vi "imp_test_v11_p2.vi"() -> ()   [LabVIEW 2014]
uses:
  <vilib>/LabVIEW Targets/FPGA/cRIO/shared/nicrio_ModuleControls/nicrio_cRIO-9237_DataRatesRing.ctl
  <vilib>/LabVIEW Targets/FPGA/cRIO/shared/nicrio_ModuleControls/nicrio_cRIO-9237_ExcitationVoltageRing.ctl
  <vilib>/rvi/FXPMathLib/FxpSinAndCos/subVIs/nifxpmath_SinAndCos_SimConfig.ctl
  <vilib>/rvi/Emulation/niFpgaGetClockAttributes.vi
  <vilib>/rvi/Emulation/niFpgaSctlEmulationGetInTimedLoop.vi
  <vilib>/rvi/Emulation/niFpgaEmulationReportErrorSimple.vi
  <vilib>/rvi/Emulation/niFpgaProcessEmulError.vi
  <vilib>/rvi/interface/RandomDataEmulation/nirviRandomDataMultiElementFPGAFIFO.vi
  <instcachedir>/0/nirviRandomDataMultiElementFPGAFIFO_AD0CFC12EF974623A9C2E4184BC062B2.lvgen/nirviRandomDataMultiElementFPGAFIFO_AD0CFC12EF974623A9C2E4184BC062B2_028.vi
  <vilib>/rvi/interface/RandomDataEmulation/niFpgaRandomDataHandleErrors.vi
  <vilib>/rvi/Emulation/niFpgaCriticalErrorInLSC.vi
  <vilib>/rvi/FXPMathLib/FxpSinAndCos/simVIs/DllFxpSinAndCosTemp_sub.vi
  <vilib>/rvi/eio/common/nirviEmuTemplateMethod_errors.vi
  <vilib>/rvi/eio/common/nirviEmuTemplatePropertySet_errors.vi
  <vilib>/rvi/DataTransferAndStorage/Container/XNode/niFpgaContainer.xnode
  <vilib>/rvi/interface/RandomDataEmulation/nirviRandomDataFpgaMultiElementTemplate.vi
  <vilib>/rvi/Analysis/measure/butterworth/XNode/niFpgaButterworthFilter.xnode
  <vilib>/rvi/FXPMathLib/FxpSinAndCos/XNode/nifxpmath_SinAndCos.xnode
  <vilib>/eio/EIONode/EIONode.xnode
  <vilib>/eio/EIOPropertyNode/EIOPropertyNode.xnode
  <vilib>/rvi/eio/common/nirviEmuTemplatePropertyGet_errors.vi
  <vilib>/rvi/eio/common/nirviEmuTemplatePropertyGet_noerrors.vi
  <vilib>/rvi/eio/common/nirviEmuTemplatePropertySet_noerrors.vi
panel:
  in  "Mavg f loop(uSec)":u32
  in  "F_Threshold_p":fxp<+,12,4>
  out "omega_p (Mavg)":fxp<+/-,36,13>
  out "Dp_d (Mavg)":fxp<+/-,36,13>
  out "omega_p2 (Mavg)":fxp<+/-,36,14>
  out "Dp2_d (Mavg)":fxp<+/-,36,14>
  in  "mt0_p2":u32
  out "Dp_d (Mavg w. f.)":fxp<+/-,36,14>
  in  "Dp_d (Mavg) coeff.":i32[](array[numeric])=[946630756, 63555534]
  out "omega_p (Mavg w. f)":fxp<+/-,36,14>
  in  "omega_P(Mavg) coeff.":i32[](array[numeric])=[946630756, 63555534]
  out "PID (kHz)":fxp<+/-,20,10>
  in  "Set 6":bool
  in  "Set 5":bool
  in  "Set 4":bool
  in  "Set 3":bool
  in  "Set 2":bool
  in  "Set 1":bool
  out "Dp1_d (T)":fxp<+/-,36,13>
  out "omega_p1 (T)":fxp<+/-,36,13>
  out "Dp2_d (T)":fxp<+/-,36,13>
  out "omega_p2 (T)":fxp<+/-,36,13>
  out "mt_omega_p2":u32
  out "Encoder Position_p2":i32
  out "D_p2":fxp<+/-,32,7>
  out "rad_p2":fxp<+/-,33,20>
  out "D_p1":fxp<+/-,32,7>
  out "rad_p1":fxp<+/-,33,20>
  out "Encoder Position_p1":i32
  out "Dp1_d (Mavg)":fxp<+/-,36,14>
  out "omega_p1 (Mavg)":fxp<+/-,36,14>
  in  "Dp_d_M_avg_Tc (uSec)":i32
  out "Dp_d (T)":fxp<+/-,36,13>
  out "omega_p (T)":fxp<+/-,36,13>
  in  "Vp. Est.":i16(ring) items=["T", "Mavg", "Mavg w. f."]
  in  "Mag. factor_p":fxp<+/-,20,3>
  in  "Mag. encoder_p":bool
  in  "Belt_out_p":fxp<+/-,7,7>
  in  "Belt_in_p":fxp<+/-,6,6>
  out "Fp_dc":fxp<+/-,32,10>
  in  "Zero_p":bool
  in  "mt0_p1":u32
  in  "Encoder reset":bool
  out "fpt_d":fxp<+/-,36,18>
  out "Dp_error_dd":fxp<+/-,36,16>
  out "Dp_error_d":fxp<+/-,33,8>
  in  "Dp_dd coeff.":i32[](array[numeric])=[946630756, 63555534]
  out "Dp_dd":fxp<+/-,36,25>
  out "dFp_PID":fxp<+/-,36,18>
  in  "dFp_PID coeff.":i32[](array[numeric])=[946630756, 63555534]
  out "fpt_i":fxp<+/-,34,18>
  in  "Bv_p":fxp<+/-,22,8>
  in  "Kv_p":fxp<+/-,26,7>
  out "Dp_error":fxp<+/-,22,7>
  out "Dpr_sin":fxp<+/-,22,7>
  in  "Sin offset_p":fxp<+/-,22,7>
  in  "Sin magnitude_p":fxp<+/-,21,6>
  out "Dpr_sin_dd":fxp<+/-,35,20>
  out "Dpr_sin_d":fxp<+/-,33,15>
  out "Sin omega_p":fxp<+/-,34,9>
  in  "Sin wave freq._p (Hz)":fxp<+/-,32,6>
  in  "Dpr_step":fxp<+/-,22,7>
  out "Dpr_for":fxp<+/-,22,7>
  in  "Command_p":i16(ring) items=["Step", "Sine"]
  in  "Ki_p":fxp<+/-,30,9>
  out "Fp_PID":fxp<+/-,36,16>
  in  "fp_tolorance":fxp<+,22,6>
  out "fp_tilde":fxp<+/-,33,10>
  in  "Kd_p":fxp<+/-,30,9>
  in  "Kp_p":fxp<+/-,32,13>
  out "Fr_p":fxp<+/-,32,10>
  in  "S/F coeff_p":fxp<+/-,25,-10>
  out "va_p":fxp<+/-,36,7>
  out "vb_p":fxp<+/-,37,8>
  out "vq_p_F":fxp<+/-,20,5> format="%.57g"
  out "vd_p_F":fxp<+/-,20,5>
  in  "dFp_add":bool
  in  "Stop motor_p":bool
  out "Force_p":fxp<+/-,32,10>
  in  "Strain selection_p":i16(ring) items=["Raw", "Avg.8", "Avg.8 w. filter"]
  out "Strain_p (Avg8 w. f)":fxp<+/-,36,8>
  in  "Strain_p Avg.8 coeff.":i32[](array[numeric])=[946630756, 63555534]
  out "Strain_p (Avg8)":fxp<+/-,36,4>
  out "Raw Strain_p":fxp<+/-,36,4>
  out "Mod6/AI3":fxp<+/-,36,4>
  in  "Strain gage reset_p":bool
  out "Dp_d (mm/s)":fxp<+/-,36,13>
  out "omega_p (rad/s)":fxp<+/-,36,13>
  out "mt_omega_p1":u32
  out "rad_p(NrTheta)":fxp<+/-,33,20>
  out "D_p(mm)":fxp<+/-,32,7>
  out "Encoder Position_p":i32
  in  "Encoder reset_p":bool
  out "Time now(s)":fxp<+,52,14>
  in  "Drive mode":i16(ring) items=["Backward", "Forward", "Imp"]
  in  "Ini coe.":bool
  out "Loop rate (kHz)":fxp<+/-,36,7>
  in  "Stop (Strain)":bool
  in  "Excitation Voltage":T1 items=["2.5 Volts", "3.3 Volts", "5.0 Volts", "10.0 Volts", "External Excitation"]
  in  "Data Rate":T2=1 items=["50.000 kS/s (NI 9237)"=1, "25.000 kS/s (NI 9237)"=2, "16.667 kS/s (NI 9237)"=3, "12.500 kS/s (NI 9237)"=4, "10.000 kS/s (NI 9237)"=5, "8.333 kS/s (NI 9237)"=6, "7.143 kS/s (NI 9237)"=7, "6.250 kS/s (NI 9237)"=8, "5.556 kS/s (NI 9237)"=9, "5.000 kS/s (NI 9237)"=10, "4.545 kS/s (NI 9237)"=11, "4.167 kS/s (NI 9237)"=12, "3.846 kS/s (NI 9237)"=13, "3.571 kS/s (NI 9237)"=14, "3.333 kS/s (NI 9237)"=15, "3.125 kS/s (NI 9237)"=16, "2.941 kS/s (NI 9237)"=17, "2.778 kS/s (NI 9237)"=18, "2.632 kS/s (NI 9237)"=19, "2.500 kS/s (NI 9237)"=20, "2.381 kS/s (NI 9237)"=21, "2.273 kS/s (NI 9237)"=22, "2.174 kS/s (NI 9237)"=23, "2.083 kS/s (NI 9237)"=24, "2.000 kS/s (NI 9237)"=25, "1.923 kS/s (NI 9237)"=26, "1.852 kS/s (NI 9237)"=27, "1.786 kS/s (NI 9237)"=28, "1.724 kS/s (NI 9237)"=29, "1.667 kS/s (NI 9237)"=30, "1.613 kS/s (NI 9237)"=31]
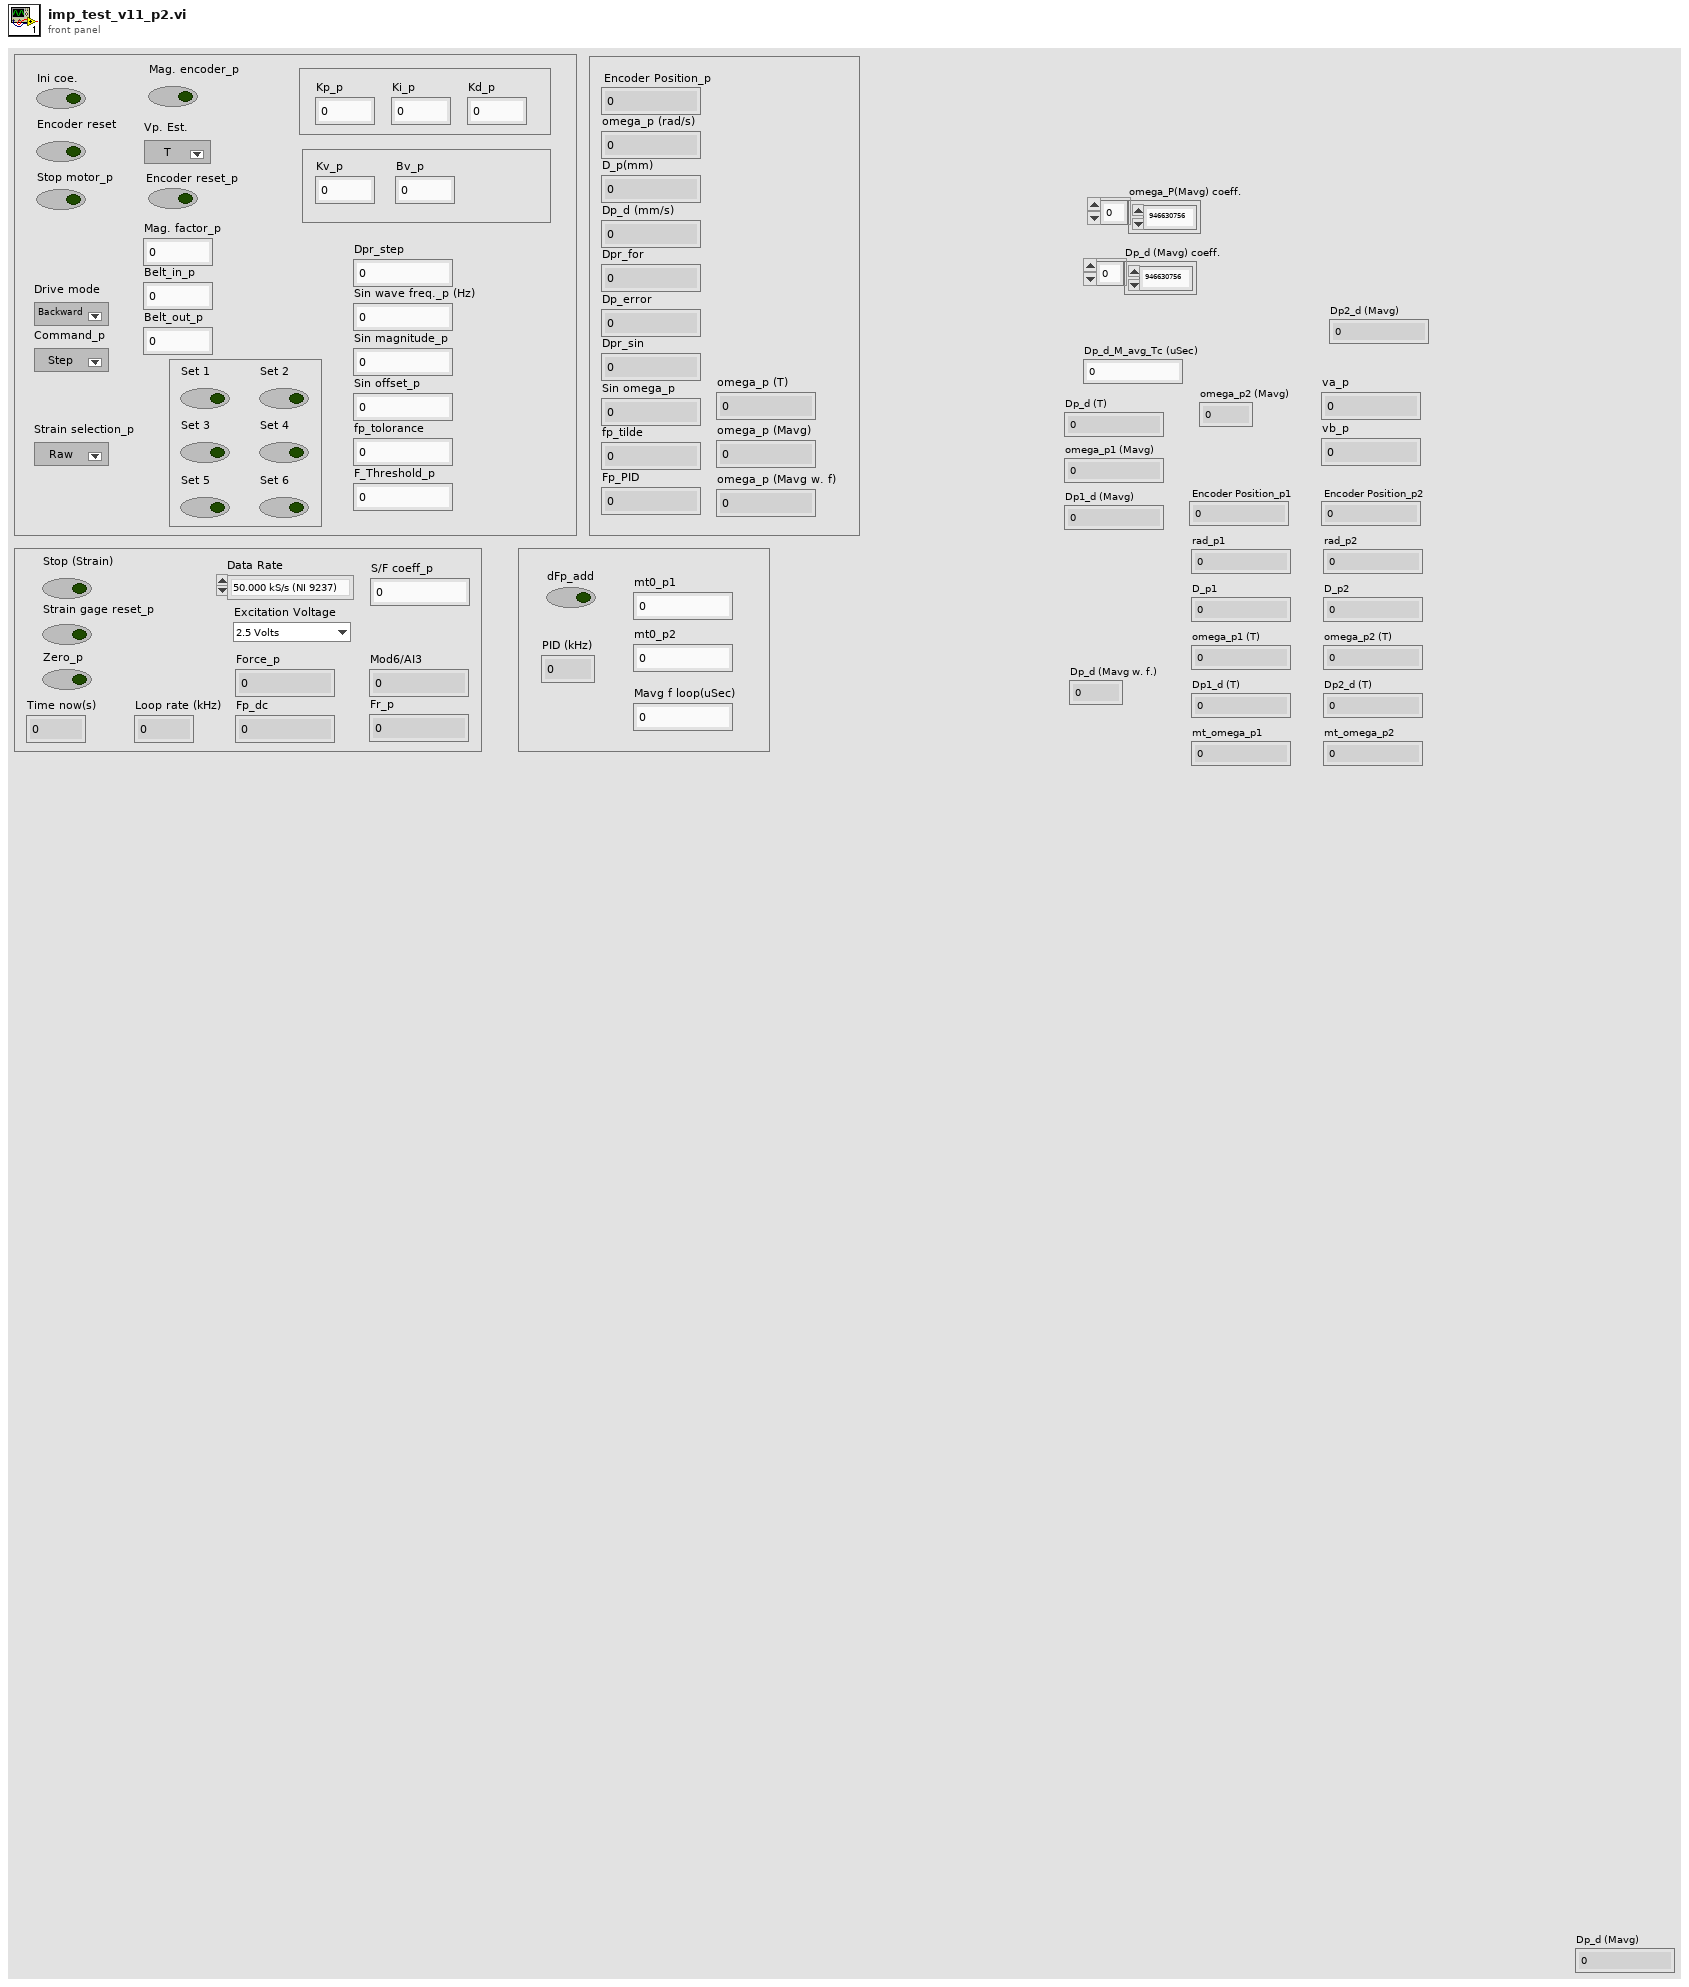
[diagram p1: front panel]
types:
  T1 = typedef "nicrio_cRIO-9237_ExcitationVoltageRing.ctl" = u8
  T2 = typedef "nicrio_cRIO-9237_DataRatesRing.ctl" = u8
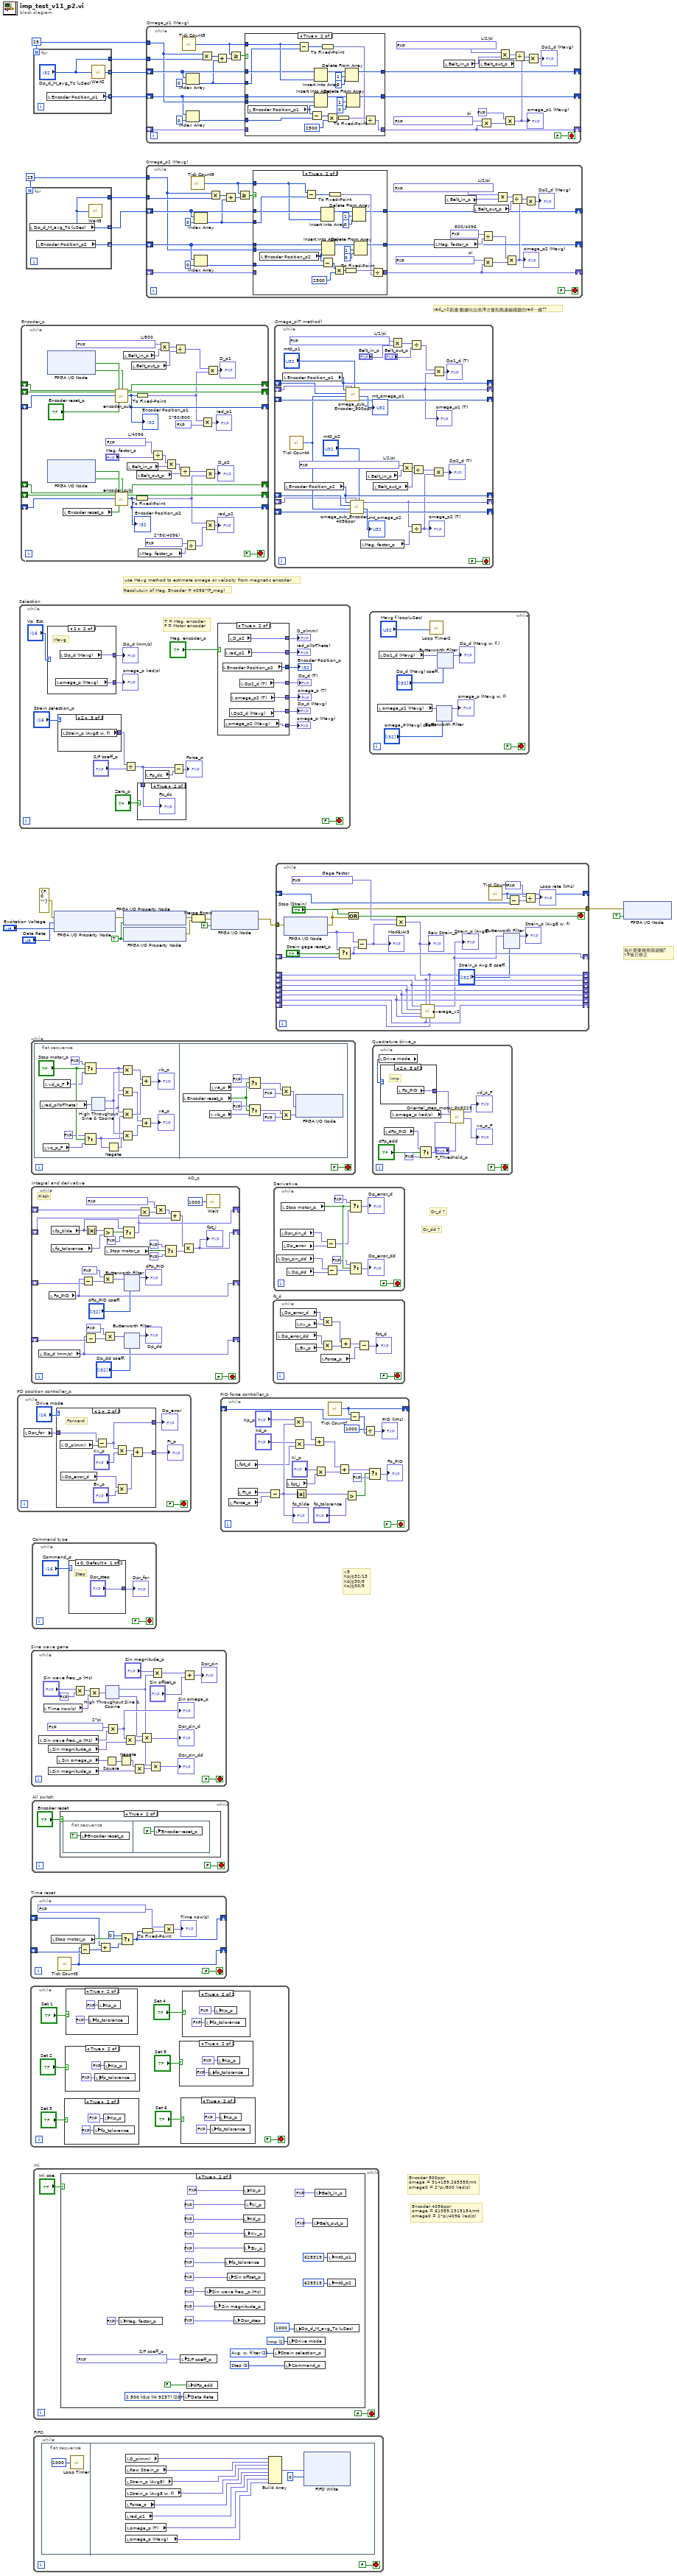
[diagram p0: block diagram]
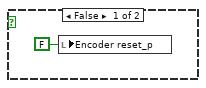
[diagram p10: hidden frame]
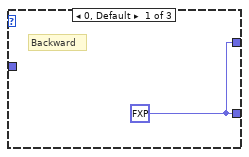
[diagram p11: hidden frame]
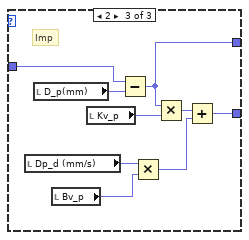
[diagram p12: hidden frame]
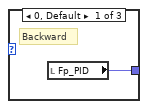
[diagram p13: hidden frame]
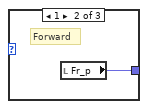
[diagram p14: hidden frame]
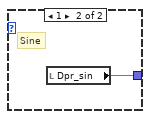
[diagram p15: hidden frame]
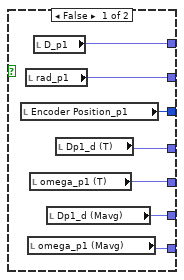
[diagram p16: hidden frame]
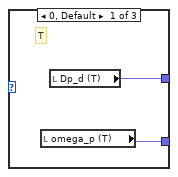
[diagram p17: hidden frame]
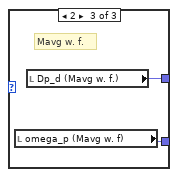
[diagram p18: hidden frame]
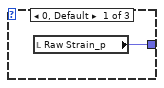
[diagram p20: hidden frame]
diagram:
  w2 = 25
  w8 = 25
  w13 = TRUE ("Half-Bridge Enable")
  # "rad_x2那邊:數據叫出來/8才會和馬達編碼器的rad一樣??"
  # "Encoder 4096ppr\nomega = 61359.2315154/mt\nomega0 = 2*pi/4096 (rad/s)"
  # "Encoder 800ppr\nomega = 314159.265359/mt\nomega0 = 2*pi/800 (rad/s)"
  # "v9\nKp改32/13\nKd改30/9\nKo改30/9"
  # "Resolutuin of Mag. Encoder = 4096*(F_mag)"
  # "use Mavg method to estimate omega or velocity from magnetic encoder"
  # "為什麼要寫兩個迴圈?\nv9後已修正"
  # "Dr_dd ?"
  # "Dr_d ?"
  n1 = while "PD position controller_p" {
    stop <- FALSE stop-if-true
    n2 = local read "Dpr_for"() -> (w21:fxp<+/-,22,7>)
    n3 = case shown="1" "Drive mode" {
      tunnel: [w26 w30 w37] -> w25
      tunnel: [w26 w28 w42] -> w22
      tunnel: w21 -> [_ w27 w36]
      frame 0, Default {
        w26 = fxp<+/-,62,19> 0.0
        # "Backward"
      }
      frame 1 {
        # "Forward"
        n4 = local read "D_p(mm)"() -> (w35:fxp<+/-,32,7>)
        n5 = local read "Dp_error_d"() -> (w29:fxp<+/-,33,8>)
        n6 = Subtract(x=w27, y=w35) -> (x-y=w28:fxp<+/-,33,8>)
        n7 = Multiply(x=w28, y="Kv_p") -> (x*y=w32:fxp<+/-,58,14>)
        n8 = Multiply(x=w29, y="Bv_p") -> (x*y=w31:fxp<+/-,55,16>)
        n9 = Add(x=w32, y=w31) -> (x+y=w30:fxp<+/-,60,16>)
      }
      frame 2 {
        # "Imp"
        n10 = local read "Dp_d (mm/s)"() -> (w40:fxp<+/-,36,13>)
        n11 = local read "D_p(mm)"() -> (w43:fxp<+/-,32,7>)
        n12 = local read "Bv_p"() -> (w39:fxp<+/-,22,8>)
        n13 = local read "Kv_p"() -> (w44:fxp<+/-,26,7>)
        n14 = Subtract(x=w36, y=w43) -> (x-y=w42:fxp<+/-,33,8>)
        n15 = Multiply(x=w40, y=w39) -> (x*y=w38:fxp<+/-,58,21>)
        n16 = Multiply(x=w42, y=w44) -> (x*y=w41:fxp<+/-,58,14>)
        n17 = Add(x=w41, y=w38) -> (x+y=w37:fxp<+/-,64,21>)
      }
    }
    "Fr_p" <- w25
    "Dp_error" <- w22
  }
  n18 = while "Selection" {
    stop <- FALSE stop-if-true
    # "T = Mag. encoder\nF = Motor encoder"
    n19 = case shown="1" "Vp. Est." {
      tunnel: [w79 w80 w83] -> w55
      tunnel: [w78 w81 w82] -> w56
      frame 0, Default {
        # "T"
        n20 = local read "omega_p (T)"() -> (w79:fxp<+/-,36,13>)
        n21 = local read "Dp_d (T)"() -> (w78:fxp<+/-,36,13>)
      }
      frame 1 {
        # "Mavg"
        n22 = local read "omega_p (Mavg)"() -> (w80:fxp<+/-,36,13>)
        n23 = local read "Dp_d (Mavg)"() -> (w81:fxp<+/-,36,13>)
      }
      frame 2 {
        # "Mavg w. f."
        n24 = local read "omega_p (Mavg w. f)"() -> (w83:fxp<+/-,36,14>)
        n25 = local read "Dp_d (Mavg w. f.)"() -> (w82:fxp<+/-,36,14>)
      }
    }
    "Dp_d (mm/s)" <- w56
    "omega_p (rad/s)" <- w55
    n26 = case shown="2" "Strain selection_p" {
      tunnel: [w85 w86 w87] -> w62
      frame 0, Default {
        n27 = local read "Raw Strain_p"() -> (w85:fxp<+/-,36,4>)
      }
      frame 1 {
        n28 = local read "Strain_p (Avg8)"() -> (w86:fxp<+/-,36,4>)
      }
      frame 2 {
        n29 = local read "Strain_p (Avg8 w. f)"() -> (w87:fxp<+/-,36,8>)
      }
    }
    n30 = Divide(x=w62, y="S/F coeff_p") -> (x/y=w59:fxp<+/-,32,10>)
    n31 = case shown="True" "Zero_p" {
      tunnel: w59 -> [_ w84]
      frame False {
      }
      frame True {
        "Fp_dc" <- w84
      }
    }
    n32 = local read "Fp_dc"() -> (w57:fxp<+/-,32,10>)
    n33 = Subtract(x=w59, y=w57) -> (x-y=→"Force_p":fxp<+/-,33,11>)
    n34 = case shown="True" "Mag. encoder_p" {
      tunnel: [w70 w77] -> w51
      tunnel: [w69 w76] -> w52
      tunnel: [w68 w75] -> w53
      tunnel: [w66 w74] -> w49
      tunnel: [w67 w73] -> w48
      tunnel: [w65 w71] -> w47
      tunnel: [w64 w72] -> w46
      frame False {
        n35 = local read "Encoder Position_p1"() -> (w68:i32)
        n36 = local read "rad_p1"() -> (w69:fxp<+/-,33,20>)
        n37 = local read "omega_p1 (Mavg)"() -> (w64:fxp<+/-,36,14>)
        n38 = local read "omega_p1 (T)"() -> (w66:fxp<+/-,36,13>)
        n39 = local read "D_p1"() -> (w70:fxp<+/-,32,7>)
        n40 = local read "Dp1_d (Mavg)"() -> (w65:fxp<+/-,36,14>)
        n41 = local read "Dp1_d (T)"() -> (w67:fxp<+/-,36,13>)
      }
      frame True {
        n42 = local read "Encoder Position_p2"() -> (w75:i32)
        n43 = local read "omega_p2 (Mavg)"() -> (w72:fxp<+/-,36,14>)
        n44 = local read "rad_p2"() -> (w76:fxp<+/-,33,20>)
        n45 = local read "D_p2"() -> (w77:fxp<+/-,32,7>)
        n46 = local read "Dp2_d (Mavg)"() -> (w71:fxp<+/-,36,14>)
        n47 = local read "omega_p2 (T)"() -> (w74:fxp<+/-,36,13>)
        n48 = local read "Dp2_d (T)"() -> (w73:fxp<+/-,36,13>)
      }
    }
    "D_p(mm)" <- w51
    "rad_p(NrTheta)" <- w52
    "Encoder Position_p" <- w53
    "Dp_d (T)" <- w48
    "omega_p (T)" <- w49
    "Dp_d (Mavg)" <- w47
    "omega_p (Mavg)" <- w46
  }
  n49 = while "Encoder_p" {
    shift-right: [w125] -> _
    shift-left: _ -> [w124]
    shift-right: [w126] -> _
    shift-left: _ -> [w123]
    shift-right: [w120] -> _
    shift-left: _ -> [w122]
    shift-right: [w111] -> _
    shift-left: _ -> [w110]
    shift-right: [w112] -> _
    shift-left: _ -> [w113]
    shift-right: [w107] -> _
    shift-left: _ -> [w108]
    stop <- FALSE stop-if-true
    w103 = fxp<+/-,20,-5> 0.00048828125  # L/4096
    w101 = fxp<+/-,16,1> 0.0244140625  # 2*50/4096)
    w119 = fxp<+/-,20,-5> 0.002499997615814209  # L/800
    w93 = fxp<+/-,16,1> 0.125  # 2*50/800
    n50 = xnode "FPGA I/O Node"() -> ("Mod7/DIO0"=w128:bool, "Mod7/DIO1"=w127:bool)  [unwired: 2 in, 2 out]
    n51 = xnode "FPGA I/O Node"() -> ("Mod7/DIO4"=w115:bool, "Mod7/DIO5"=w114:bool)  [unwired: 2 in, 2 out]
    n52 = local read "Encoder reset_p"() -> (w109:bool)
    n53 = call "encoder_sub.vi"("A_pre"=w124, "B_pre"=w123, "Encoder Position_pre"=w122, "A input"=w128, "Encoder Position Reset"="Encoder reset_p", "B input"=w127) -> ("A"=w125:bool, "B"=w126:bool, "Encoder Position (Counts)"=w120:i32)  [unwired: 19 in]
    "Encoder Position_p1" <- w120
    n54 = call "encoder_sub.vi"("A_pre"=w110, "B_pre"=w113, "Encoder Position_pre"=w108, "A input"=w115, "Encoder Position Reset"=w109, "B input"=w114) -> ("A"=w111:bool, "B"=w112:bool, "Encoder Position (Counts)"=w107:i32)  [unwired: 19 in]
    "Encoder Position_p2" <- w107
    n55 = local read "Belt_in_p"() -> (w118:fxp<+/-,6,6>)
    n56 = local read "Belt_in_p"() -> (w104:fxp<+/-,6,6>)
    n57 = local read "Belt_out_p"() -> (w116:fxp<+/-,7,7>)
    n58 = To Fixed-Point(number=w107) -> (fixed-point=w89:fxp<+/-,32,32>)  [unwired: 1 in]
    n59 = To Fixed-Point(number=w120) -> (fixed-point=w94:fxp<+/-,32,32>)  [unwired: 1 in]
    n60 = local read "Belt_out_p"() -> (w106:fxp<+/-,7,7>)
    n61 = local read "Mag. factor_p"() -> (w100:fxp<+/-,20,3>)
    n62 = Divide(x=w103, y="Mag. factor_p") -> (x/y=w102:fxp<+/-,41,13>)
    n63 = Multiply(x=w119, y=w118) -> (x*y=w117:fxp<+/-,26,1>)
    n64 = Multiply(x=w102, y=w104) -> (x*y=w105:fxp<+/-,46,18>)
    n65 = Divide(x=w117, y=w116) -> (x/y=w96:fxp<+/-,33,1>)
    n66 = Divide(x=w105, y=w106) -> (x/y=w91:fxp<+/-,53,18>)
    n67 = Divide(x=w101, y=w100) -> (x/y=w88:fxp<+/-,37,5>)
    n68 = Multiply(x=w94, y=w93) -> (x*y=→"rad_p1":fxp<+/-,33,20>)
    n69 = Multiply(x=w91, y=w89) -> (x*y=→"D_p2":fxp<+/-,37,7>)
    n70 = Multiply(x=w89, y=w88) -> (x*y=→"rad_p2":fxp<+/-,46,16>)
    n71 = Multiply(x=w96, y=w94) -> (x*y=→"D_p1":fxp<+/-,32,7>)
  }
  n72 = for {
    N: w2 -> [_]
    tunnel: [w130] -> w4 mode=indexing
    tunnel: [w129] -> w3 mode=indexing
    tunnel: [w129] -> w1
    n73 = local read "Dp_d_M_avg_Tc (uSec)"() -> (w129:i32)
    n74 = local read "Encoder Position_p2"() -> (w130:i32)
    n75 = call "Wait5"("Count(uSec)"=w129) -> ()  [unwired: 1 out]
  }
  n76 = while "Time reset" {
    shift-right: [w140] -> _
    shift-left: _ -> [w141]
    shift-right: [w135] -> _
    shift-left: _ -> [w136]
    stop <- FALSE stop-if-true
    n77 = local read "Stop motor_p"() -> (w142:bool)
    n78 = call "Tick Count3"() -> ("Tick Count(uSec)"=w140:u32)
    n79 = Subtract(x=w140, y=w141) -> (x-y=w139:u32)
    n80 = Add(x=w136, y=w139) -> (x+y=w138:u32)
    n81 = Select(t=u32 0, s=w142, f=w138) -> (s? t:f=w135:u32)
    n82 = To Fixed-Point(number=w135) -> (fixed-point=w134:fxp<+,32,32>)  [unwired: 1 in]
    n83 = Multiply(x=fxp<+,20,-18> 1.0000003385357559e-06, y=w134) -> (x*y=→"Time now(s)":fxp<+,52,14>)
  }
  n84 = while {
    stop <- FALSE stop-if-true
    n85 = case shown="True" "Set 3" {
      frame False {
      }
      frame True {
        n86 = local write "fp_tolorance"(fxp<+,22,6> 3.0 ("fp_tolorance")) -> ()
        n87 = local write "Kp_p"(fxp<+/-,36,9> 100.0 ("Kp_p")) -> ()
      }
    }
    n88 = case shown="True" "Set 2" {
      frame False {
      }
      frame True {
        n89 = local write "fp_tolorance"(fxp<+,22,6> 1.5 ("fp_tolorance")) -> ()
        n90 = local write "Kp_p"(fxp<+/-,36,9> 50.0 ("Kp_p")) -> ()
      }
    }
    n91 = case shown="True" "Set 1" {
      frame False {
      }
      frame True {
        n92 = local write "fp_tolorance"(fxp<+,22,6> 3.0 ("fp_tolorance")) -> ()
        n93 = local write "Kp_p"(fxp<+/-,36,9> 50.0 ("Kp_p")) -> ()
      }
    }
    n94 = case shown="True" "Set 5" {
      frame False {
      }
      frame True {
        n95 = local write "fp_tolorance"(fxp<+,22,6> 3.0 ("fp_tolorance")) -> ()
        n96 = local write "Kp_p"(fxp<+/-,36,9> 150.0 ("Kp_p")) -> ()
      }
    }
    n97 = case shown="True" "Set 6" {
      frame False {
      }
      frame True {
        n98 = local write "fp_tolorance"(fxp<+,22,6> 1.5 ("fp_tolorance")) -> ()
        n99 = local write "Kp_p"(fxp<+/-,36,9> 150.0 ("Kp_p")) -> ()
      }
    }
    n100 = case shown="True" "Set 4" {
      frame False {
      }
      frame True {
        n101 = local write "fp_tolorance"(fxp<+,22,6> 1.5 ("fp_tolorance")) -> ()
        n102 = local write "Kp_p"(fxp<+/-,36,9> 100.0 ("Kp_p")) -> ()
      }
    }
  }
  n103 = while "AO_p" {
    stop <- FALSE stop-if-true
    n104 = flat-sequence {
      frame #0 {
        n105 = local read "rad_p(NrTheta)"() -> (w174:fxp<+/-,33,20>)
        n106 = local read "vq_p_F"() -> (w175:fxp<+/-,20,5>)
        n107 = local read "vd_p_F"() -> (w177:fxp<+/-,20,5>)
        n108 = Select(t=fxp<+/-,20,5> 0.0, s="Stop motor_p", f=w177) -> (s? t:f=w166:fxp<+/-,20,5>)
        n109 = Select(t=fxp<+,1,1> 0.0, s="Stop motor_p", f=w175) -> (s? t:f=w165:fxp<+/-,20,5>)
        n110 = xnode "High Throughput Sine & Cosine"("x (pi)"=w174) -> ("sin(x)"=w168:fxp<+/-,16,2>, "cos(x)"=w167:fxp<+/-,16,2>)
        n111 = Negate(x=w165) -> (-x=w173:fxp<+/-,21,6>)
        n112 = Multiply(x=w166, y=w168) -> (x*y=w172:fxp<+/-,36,7>)
        n113 = Multiply(x=w166, y=w167) -> (x*y=w170:fxp<+/-,36,7>)
        n114 = Multiply(x=w167, y=w165) -> (x*y=w171:fxp<+/-,36,7>)
        n115 = Multiply(x=w168, y=w173) -> (x*y=w169:fxp<+/-,35,6>)
        n116 = Add(x=w172, y=w171) -> (x+y=→"vb_p":fxp<+/-,37,8>)
        n117 = Add(x=w170, y=w169) -> (x+y=→"va_p":fxp<+/-,36,7>)
      }
      frame #1 {
        n118 = local read "Encoder reset_p"() -> (w210:bool)
        n119 = local read "vb_p"() -> (w211:fxp<+/-,37,8>)
        n120 = local read "va_p"() -> (w212:fxp<+/-,36,7>)
        n121 = Select(t=fxp<+,2,2> 3.0, s=w210, f=w212) -> (s? t:f=w218:fxp<+/-,36,7>)
        n122 = Select(t=fxp<+,1,1> 0.0, s=w210, f=w211) -> (s? t:f=w217:fxp<+/-,37,8>)
        n123 = Multiply(x=w218, y=fxp<+/-,1,0> -0.5) -> (x*y=w213:fxp<+/-,36,6>)
        n124 = Multiply(x=w217, y=fxp<+/-,1,0> -0.5) -> (x*y=w214:fxp<+/-,36,6>)
        n125 = xnode "FPGA I/O Node"("Mod8/AO0"=w213, "Mod8/AO1"=w214) -> ()  [unwired: 2 in, 2 out]
      }
    }
  }
  n126 = while "Sine wave gene" {
    stop <- FALSE stop-if-true
    w226 = fxp<+,20,3> 6.2831878662109375  # 2*pi
    n127 = local read "Sin wave freq._p (Hz)"() -> (w222:fxp<+/-,32,6>)
    n128 = local read "Time now(s)"() -> (w240:fxp<+,52,14>)
    n129 = local read "Sin magnitude_p"() -> (w223:fxp<+/-,21,6>)
    n130 = local read "Sin magnitude_p"() -> (w225:fxp<+/-,21,6>)
    n131 = local read "Sin omega_p"() -> (w224:fxp<+/-,34,9>)
    n132 = Multiply(x="Sin wave freq._p (Hz)", y=fxp<+/-,10,3> 2.0) -> (x*y=w244:fxp<+/-,42,9>)
    n133 = Multiply(x=w244, y=w240) -> (x*y=w241:fxp<+/-,41,19>)
    n134 = Square(x=w224) -> (x^2=w236:fxp<+,34,18>)
    n135 = xnode "High Throughput Sine & Cosine"("x (pi)"=w241) -> ("sin(x)"=w227:fxp<+/-,16,2>, "cos(x)"=w232:fxp<+/-,16,2>)
    n136 = Multiply(x=w226, y=w222) -> (x*y=w239:fxp<+/-,34,9>)
    "Sin omega_p" <- w239
    n137 = Negate(x=w236) -> (-x=w235:fxp<+/-,35,19>)
    n138 = Multiply(x=w239, y=w223) -> (x*y=w238:fxp<+/-,33,15>)
    n139 = Multiply(x=w235, y=w225) -> (x*y=w234:fxp<+/-,35,19>)
    n140 = Multiply(x=w232, y=w238) -> (x*y=→"Dpr_sin_d":fxp<+/-,33,15>)
    n141 = Multiply(x=w227, y=w234) -> (x*y=→"Dpr_sin_dd":fxp<+/-,35,20>)
    n142 = Multiply(x="Sin magnitude_p", y=w227) -> (x*y=w230:fxp<+/-,37,8>)
    n143 = Add(x=w230, y="Sin offset_p") -> (x+y=→"Dpr_sin":fxp<+/-,37,8>)
  }
  n144 = while "Integral and derivative" {
    shift-right: [w298] -> _
    shift-left: _ -> [w301]
    shift-right: [w291] -> _
    shift-left: _ -> [w290]
    shift-right: [w285] -> _
    shift-left: _ -> [w284]
    shift-right: [w280] -> _
    shift-left: _ -> [w281]
    stop <- FALSE stop-if-true
    # "Pitch"
    n145 = local read "Dp_d (mm/s)"() -> (w280:fxp<+/-,36,13>)
    n146 = local read "Fp_PID"() -> (w285:fxp<+/-,36,16>)
    n147 = local read "fp_tilde"() -> (w302:fxp<+/-,33,10>)
    n148 = local read "fp_tolorance"() -> (w305:fxp<+,22,6>)
    n149 = Subtract(x=w285, y=w284) -> (x-y=w289:fxp<+/-,37,17>)
    n150 = Subtract(x=w280, y=w281) -> (x-y=w282:fxp<+/-,37,14>)
    n151 = Absolute Value(x=w302) -> (abs(x)=w306:fxp<+,33,10>)
    n152 = Greater?(x=w306, y=w305) -> (0:w304:bool)
    n153 = Multiply(x=fxp<+,7,10> 1000.0, y=w289) -> (x*y=w287:fxp<+/-,32,18>)
    n154 = Multiply(x=fxp<+,7,10> 1000.0, y=w282) -> (x*y=w278:fxp<+/-,36,21>)
    n155 = local read "Stop motor_p"() -> (w293:bool)
    n156 = Select(t=w302, s=w304, f=fxp<+,1,1> 0.0) -> (s? t:f=w298:fxp<+/-,33,10>)
    n157 = xnode "Butterworth Filter"("input data"=w287, "scaled coefficients"="dFp_PID coeff.") -> ("output data"=→"dFp_PID":fxp<+/-,36,22>)  [unwired: 1 in]
    n158 = xnode "Butterworth Filter"("input data"=w278, "scaled coefficients"="Dp_dd coeff.") -> ("output data"=→"Dp_dd":fxp<+/-,36,25>)  [unwired: 1 in]
    n159 = Multiply(x=w301, y=w298) -> (x*y=w300:fxp<+/-,34,12>)
    n160 = Multiply(x=fxp<+/-,30,12> 0.000499725341796875, y=w300) -> (x*y=w297:fxp<+/-,34,10>)
    n161 = Select(t=fxp<+,1,1> 0.0, s=w293, f=fxp<+,1,1> 1.0) -> (s? t:f=w295:fxp<+,1,1>)
    n162 = Add(x=w297, y=w290) -> (x+y=w296:fxp<+/-,36,16>)
    n163 = Multiply(x=w296, y=w295) -> (x*y=w291:fxp<+/-,34,18>)
    "fpt_i" <- w291
    n164 = call "Wait"("Count(uSec)"=u32 1000) -> ()  [unwired: 1 out]
  }
  n165 = while "Command type" {
    stop <- FALSE stop-if-true
    n166 = case shown="0, Default" "Command_p" {
      tunnel: ["Dpr_step" w328] -> w325
      frame 0, Default {
        # "Step"
      }
      frame 1 {
        # "Sine"
        n167 = local read "Dpr_sin"() -> (w328:fxp<+/-,22,7>)
      }
    }
    "Dpr_for" <- w325
  }
  n168 = while "All switch" {
    stop <- FALSE stop-if-true
    n169 = case shown="True" "Encoder reset" {
      frame False {
        n170 = local write "Encoder reset_p"(FALSE ("Encoder reset_p")) -> ()
      }
      frame True {
        n171 = flat-sequence {
          frame #0 {
            n172 = local write "Encoder reset_p"(TRUE ("Encoder reset_p")) -> ()
          }
          frame #1 {
            n173 = local write "Encoder reset_p"(FALSE ("Encoder reset_p")) -> ()
          }
        }
      }
    }
  }
  n174 = for {
    N: w8 -> [_]
    tunnel: ["Dp_d_M_avg_Tc (uSec)"] -> w5
    tunnel: [w335] -> w7 mode=indexing
    tunnel: [w334] -> w6 mode=indexing
    n175 = local read "Encoder Position_p1"() -> (w334:i32)
    n176 = call "Wait2"("Count(uSec)"="Dp_d_M_avg_Tc (uSec)") -> ("Tick Count(uSec)"=w335:u32)
  }
  n177 = while "Ini" {
    stop <- FALSE stop-if-true
    n178 = case shown="True" "Ini coe." {
      frame False {
      }
      frame True {
        w339 = i16 2 items=["Backward", "Forward", "Imp"] ("Drive mode")
        w343 = T2 20 items=["50.000 kS/s (NI 9237)"=1, "25.000 kS/s (NI 9237)"=2, "16.667 kS/s (NI 9237)"=3, "12.500 kS/s (NI 9237)"=4, "10.000 kS/s (NI 9237)"=5, "8.333 kS/s (NI 9237)"=6, "7.143 kS/s (NI 9237)"=7, "6.250 kS/s (NI 9237)"=8, "5.556 kS/s (NI 9237)"=9, "5.000 kS/s (NI 9237)"=10, "4.545 kS/s (NI 9237)"=11, "4.167 kS/s (NI 9237)"=12, "3.846 kS/s (NI 9237)"=13, "3.571 kS/s (NI 9237)"=14, "3.333 kS/s (NI 9237)"=15, "3.125 kS/s (NI 9237)"=16, "2.941 kS/s (NI 9237)"=17, "2.778 kS/s (NI 9237)"=18, "2.632 kS/s (NI 9237)"=19, "2.500 kS/s (NI 9237)"=20, "2.381 kS/s (NI 9237)"=21, "2.273 kS/s (NI 9237)"=22, "2.174 kS/s (NI 9237)"=23, "2.083 kS/s (NI 9237)"=24, "2.000 kS/s (NI 9237)"=25, "1.923 kS/s (NI 9237)"=26, "1.852 kS/s (NI 9237)"=27, "1.786 kS/s (NI 9237)"=28, "1.724 kS/s (NI 9237)"=29, "1.667 kS/s (NI 9237)"=30, "1.613 kS/s (NI 9237)"=31] ("Data Rate")
        w358 = i16 0 items=["Step", "Sine"] ("Command_p")
        w359 = i16 2 items=["Raw", "Avg.", "Avg. w. filter"] ("Strain selection_p")
        w360 = fxp<+/-,25,-10> 5.851034075021744e-07  # S/F coeff_p
        n179 = local write "Mag. factor_p"(fxp<+/-,20,3> 1.0 ("Mag. factor_p")) -> ()
        n180 = local write "S/F coeff_p"(w360) -> ()
        n181 = local write "Data Rate"(w343) -> ()
        n182 = local write "dFp_add"(FALSE ("dFp_add")) -> ()
        n183 = local write "Sin wave freq._p (Hz)"(fxp<+/-,32,6> 1.0 ("Sin wave freq._p (Hz)")) -> ()
        n184 = local write "Sin magnitude_p"(fxp<+/-,21,6> 5.0 ("Sin magnitude_p")) -> ()
        n185 = local write "fp_tolorance"(fxp<+,22,6> 5.0 ("fp_tolorance")) -> ()
        n186 = local write "Sin offset_p"(fxp<+/-,22,7> 0.0 ("Sin offset_p")) -> ()
        n187 = local write "Dpr_step"(fxp<+/-,22,7> 0.0 ("Dpr_step")) -> ()
        n188 = local write "Kp_p"(fxp<+/-,36,9> 30.0 ("Kp_p")) -> ()
        n189 = local write "Kd_p"(fxp<+/-,36,9> 0.0 ("Kd_p")) -> ()
        n190 = local write "Kv_p"(fxp<+/-,22,8> 0.0 ("Kv_p")) -> ()
        n191 = local write "Bv_p"(fxp<+/-,22,8> 0.0 ("Bv_p")) -> ()
        n192 = local write "Ki_p"(fxp<+/-,36,9> 0.0 ("Ki_p")) -> ()
        n193 = local write "Strain selection_p"(w359) -> ()
        n194 = local write "Command_p"(w358) -> ()
        n195 = local write "Drive mode"(w339) -> ()
        n196 = local write "Dp_d_M_avg_Tc (uSec)"(u32 1000 ("D_d_M_avg_Tc (uSec)")) -> ()
        n197 = local write "Belt_out_p"(fxp<+/-,7,7> 36.0 ("Belt_op")) -> ()
        n198 = local write "Belt_in_p"(fxp<+/-,6,6> 16.0 ("Belt_mp")) -> ()
        n199 = local write "mt0_p1"(u32 628319 ("mt0_p1")) -> ()
        n200 = local write "mt0_p2"(u32 628319 ("mt0_p2")) -> ()
      }
    }
  }
  n201 = while "FIFO" {
    stop <- FALSE stop-if-true
    n202 = flat-sequence {
      frame #0 {
        n203 = call "Loop Timer"("Count(uSec)"=u32 1000) -> ()  [unwired: 1 out]
      }
      frame #1 {
        n204 = local read "D_p(mm)"() -> (w370:fxp<+/-,32,7>)
        n205 = local read "Raw Strain_p"() -> (w369:fxp<+/-,36,4>)
        n206 = local read "Strain_p (Avg8)"() -> (w368:fxp<+/-,36,4>)
        n207 = local read "Strain_p (Avg8 w. f)"() -> (w367:fxp<+/-,36,8>)
        n208 = local read "Force_p"() -> (w366:fxp<+/-,32,10>)
        n209 = local read "rad_p1"() -> (w365:fxp<+/-,33,20>)
        n210 = local read "omega_p (T)"() -> (w364:fxp<+/-,36,13>)
        n211 = local read "omega_p (Mavg)"() -> (w363:fxp<+/-,36,13>)
        n212 = Build Array(w370, w369, w368, w367, w366, w365, w364, w363) -> (w371:fxp<+/-,52,20>[])
        n213 = xnode ("FIFO Write")("Element"=w371, "Timeout"=0) -> ()  [unwired: 1 in, 2 out]
      }
    }
  }
  n214 = xnode "FPGA I/O Property Node"("error in"=errorcluster {"status"=FALSE, "code"=0, "source"=""}, "Data Rate"="Data Rate", "Excitation Voltage"="Excitation Voltage") -> ("error out"=w18:errorcluster)  [unwired: 1 in, 1 out]
  n215 = xnode "FPGA I/O Property Node"("error in"=w18, "Half-Bridge Enable"=w13) -> ("error out"=w11:errorcluster)  [unwired: 1 in, 1 out]
  n216 = xnode "FPGA I/O Property Node"("Half-Bridge Enable"=w13) -> ("error out"=w10:errorcluster)  [unwired: 2 in, 1 out]
  n217 = while "Omega_p2 (Mavg)" {
    shift-right: [w374] -> _
    shift-left: w4 -> [w395]
    shift-right: [w375] -> _
    shift-left: w3 -> [w393]
    shift-right: [w379] -> _
    shift-left: _ -> [w377]
    tunnel: w2 -> [w391]
    tunnel: w1 -> [w396]
    stop <- FALSE stop-if-true
    w380 = fxp<+/-,27,3> 3.1415926814079285  # pi
    w383 = fxp<+,32,0> 0.1953125  # 800/4096
    w388 = fxp<+/-,32,0> 0.3183098859153688  # L/2/pi
    n218 = call "Tick Count9"() -> ("Tick Count(uSec)"=w390:u32)
    n219 = Index Array(array=w393, index=0) -> (element=w392:i32)
    n220 = Index Array(array=w395, index=0) -> (element=w394:i32)
    n221 = Multiply(x=w391, y=w396) -> (x*y=w399:i32)
    n222 = Add(x=w399, y=w392) -> (x+y=w398:i32)
    n223 = Greater Or Equal?(x=w390, y=w398) -> (x >= y?=w397:bool)
    n224 = case shown="True" w397 {
      tunnel: w395 -> [w403 w418]
      tunnel: w394 -> [_ w410]
      tunnel: w393 -> [w404 w419]
      tunnel: w392 -> [_ w420]
      tunnel: w391 -> [_ w417]
      tunnel: w390 -> [_ w405]
      tunnel: [w403 w408] -> w374
      tunnel: [w404 w407] -> w375
      tunnel: [w402 w406] -> w379
      tunnel: w377 -> [w402 _]
      frame False {
      }
      frame True {
        n225 = local read "Encoder Position_p2"() -> (w409:i32)
        n226 = Subtract(x=w405, y=w420) -> (x-y=w421:u32)
        n227 = Insert Into Array(array=w419, new element=w405) -> (w423:i32[])  [unwired: 1 in]
        n228 = Subtract(x=w409, y=w410) -> (x-y=w414:i32)
        n229 = Insert Into Array(array=w418, index=w417, new element=w409) -> (w424:i32[])
        n230 = To Fixed-Point(number=w421) -> (fixed-point=w411:fxp<+,32,32>)  [unwired: 1 in]
        n231 = Multiply(x=w414, y=2500) -> (x*y=w415:i32)
        n232 = To Fixed-Point(number=w415) -> (fixed-point=w416:fxp<+/-,32,32>)  [unwired: 1 in]
        n233 = Delete From Array(array=w423, length=1, index=0) -> (array with subset deleted=w407:i32[])  [unwired: 1 out]
        n234 = Delete From Array(array=w424, length=1, index=0) -> (array with subset deleted=w408:i32[])  [unwired: 1 out]
        n235 = Divide(x=w416, y=w411) -> (x/y=w406:fxp<+/-,64,32>)
      }
    }
    n236 = local read "Mag. factor_p"() -> (w382:fxp<+/-,20,3>)
    n237 = local read "Belt_in_p"() -> (w385:fxp<+/-,6,6>)
    n238 = local read "Belt_out_p"() -> (w384:fxp<+/-,7,7>)
    n239 = Divide(x=w383, y=w382) -> (x/y=w373:fxp<+/-,32,1>)
    n240 = Multiply(x=w380, y=w379) -> (x*y=w381:fxp<+/-,64,35>)
    n241 = Multiply(x=w388, y=w385) -> (x*y=w389:fxp<+/-,38,6>)
    n242 = Multiply(x=w373, y=w381) -> (x*y=w376:fxp<+/-,64,36>)
    "omega_p2 (Mavg)" <- w376
    n243 = Divide(x=w389, y=w384) -> (x/y=w387:fxp<+/-,45,6>)
    n244 = Multiply(x=w387, y=w376) -> (x*y=→"Dp2_d (Mavg)":fxp<+/-,64,41>)
  }
  n245 = while "Omega_p1 (Mavg)" {
    tunnel: w8 -> [w445]
    shift-right: [w443] -> _
    shift-left: w7 -> [w448]
    shift-right: [w442] -> _
    shift-left: w6 -> [w444]
    shift-right: [w441] -> _
    shift-left: _ -> [w440]
    tunnel: w5 -> [w438]
    stop <- FALSE stop-if-true
    w432 = fxp<+/-,27,3> 3.1415926814079285  # pi
    w431 = fxp<+/-,32,0> 0.3183098859153688  # L/2/pi
    n246 = call "Tick Count5"() -> ("Tick Count(uSec)"=w449:u32)
    n247 = Index Array(array=w448, index=0) -> (element=w447:u32)
    n248 = Index Array(array=w444, index=0) -> (element=w446:i32)
    n249 = Multiply(x=w445, y=w438) -> (x*y=w451:i32)
    n250 = Add(x=w451, y=w447) -> (x+y=w450:u32)
    n251 = Greater Or Equal?(x=w449, y=w450) -> (x >= y?=w439:bool)
    n252 = case shown="True" w439 {
      tunnel: w449 -> [_ w472]
      tunnel: w445 -> [_ w469]
      tunnel: w448 -> [w456 w471]
      tunnel: w447 -> [_ w470]
      tunnel: w446 -> [_ w466]
      tunnel: w444 -> [w455 w468]
      tunnel: [w454 w464] -> w441
      tunnel: [w456 w463] -> w443
      tunnel: [w455 w462] -> w442
      tunnel: w440 -> [w454 _]
      frame False {
      }
      frame True {
        n253 = local read "Encoder Position_p1"() -> (w465:i32)
        n254 = Subtract(x=w472, y=w470) -> (x-y=w473:u32)
        n255 = Subtract(x=w465, y=w466) -> (x-y=w458:i32)
        n256 = Insert Into Array(array=w471, new element=w472) -> (w475:u32[])  [unwired: 1 in]
        n257 = Insert Into Array(array=w468, index=w469, new element=w465) -> (w476:i32[])
        n258 = To Fixed-Point(number=w473) -> (fixed-point=w460:fxp<+,32,32>)  [unwired: 1 in]
        n259 = Multiply(x=w458, y=2500) -> (x*y=w459:i32)
        n260 = To Fixed-Point(number=w459) -> (fixed-point=w467:fxp<+/-,32,32>)  [unwired: 1 in]
        n261 = Delete From Array(array=w475, length=1, index=0) -> (array with subset deleted=w463:u32[])  [unwired: 1 out]
        n262 = Delete From Array(array=w476, length=1, index=0) -> (array with subset deleted=w462:i32[])  [unwired: 1 out]
        n263 = Divide(x=w467, y=w460) -> (x/y=w464:fxp<+/-,64,32>)
      }
    }
    n264 = local read "Belt_in_p"() -> (w436:fxp<+/-,6,6>)
    n265 = local read "Belt_out_p"() -> (w435:fxp<+/-,7,7>)
    n266 = Multiply(x=w432, y=w441) -> (x*y=w437:fxp<+/-,64,35>)
    n267 = Multiply(x=w431, y=w436) -> (x*y=w434:fxp<+/-,38,6>)
    n268 = Multiply(x=fxp<+/-,2,2> 1.0 ("f"), y=w437) -> (x*y=w430:fxp<+/-,64,37>)
    "omega_p1 (Mavg)" <- w430
    n269 = Divide(x=w434, y=w435) -> (x/y=w429:fxp<+/-,45,6>)
    n270 = Multiply(x=w429, y=w430) -> (x*y=→"Dp1_d (Mavg)":fxp<+/-,64,42>)
  }
  n271 = Merge Errors(w11, w10) -> (w12:errorcluster)
  n272 = xnode "FPGA I/O Node"("error in"=w12, "Mod6/Start"=TRUE) -> ("error out"=w16:errorcluster)  [unwired: 1 in, 1 out]
  n273 = while "PID force controller_p" {
    shift-right: [w483] -> _
    shift-left: _ -> [w482]
    stop <- FALSE stop-if-true
    n274 = local read "Force_p"() -> (w495:fxp<+/-,32,10>)
    n275 = local read "fpt_d"() -> (w491:fxp<+/-,36,18>)
    n276 = local read "Fr_p"() -> (w496:fxp<+/-,32,10>)
    n277 = Subtract(x=w496, y=w495) -> (x-y=w493:fxp<+/-,33,11>)
    "fp_tilde" <- w493
    n278 = local read "fpt_i"() -> (w487:fxp<+/-,34,18>)
    n279 = Multiply(x="Kp_p", y=w493) -> (x*y=w489:fxp<+/-,64,23>)
    n280 = Multiply(x="Kd_p", y=w491) -> (x*y=w490:fxp<+/-,64,27>)
    n281 = Absolute Value(x=w493) -> (abs(x)=w502:fxp<+,32,10>)
    n282 = Add(x=w489, y=w490) -> (x+y=w485:fxp<+/-,64,28>)
    n283 = Multiply(x="Ki_p", y=w487) -> (x*y=w486:fxp<+/-,64,27>)
    n284 = call "Tick Count7"() -> ("Tick Count(uSec)"=w483:u32)
    n285 = Add(x=w485, y=w486) -> (x+y=w484:fxp<+/-,64,29>)
    n286 = Greater?(x=w502, y="fp_tolorance") -> (0:w499:bool)
    n287 = Subtract(x=w483, y=w482) -> (x-y=w481:u32)
    n288 = Divide(x=u32 1000, y=w481) -> (x/y=→"PID (kHz)":fxp<+/-,20,7>)
    n289 = Select(t=w484, s=w499, f=fxp<+,1,1> 0.0) -> (s? t:f=→"Fp_PID":fxp<+/-,64,29>)
  }
  n290 = while "ft_d" {
    stop <- FALSE stop-if-true
    n291 = local read "Dp_error_dd"() -> (w509:fxp<+/-,36,16>)
    n292 = local read "Dp_error_d"() -> (w511:fxp<+/-,33,8>)
    n293 = local read "Kv_p"() -> (w512:fxp<+/-,26,7>)
    n294 = local read "Bv_p"() -> (w510:fxp<+/-,22,8>)
    n295 = Multiply(x=w511, y=w512) -> (x*y=w507:fxp<+/-,59,15>)
    n296 = Multiply(x=w509, y=w510) -> (x*y=w508:fxp<+/-,58,24>)
    n297 = local read "Force_p"() -> (w505:fxp<+/-,32,10>)
    n298 = Add(x=w507, y=w508) -> (x+y=w506:fxp<+/-,64,24>)
    n299 = Subtract(x=w506, y=w505) -> (x-y=→"fpt_d":fxp<+/-,64,25>)
  }
  n300 = while "Derivative" {
    stop <- FALSE stop-if-true
    n301 = local read "Dpr_sin_dd"() -> (w521:fxp<+/-,35,20>)
    n302 = local read "Dpr_sin_d"() -> (w523:fxp<+/-,33,15>)
    n303 = local read "Stop motor_p"() -> (w519:bool)
    n304 = local read "Dp_error"() -> (w524:fxp<+/-,22,7>)
    n305 = local read "Dp_dd"() -> (w522:fxp<+/-,36,25>)
    n306 = Subtract(x=w523, y=w524) -> (x-y=w516:fxp<+/-,34,16>)
    n307 = Subtract(x=w521, y=w522) -> (x-y=w520:fxp<+/-,41,26>)
    n308 = Select(t=fxp<+,1,1> 0.0, s=w519, f=w516) -> (s? t:f=→"Dp_error_d":fxp<+/-,34,16>)
    n309 = Select(t=fxp<+/-,41,26> 0.0, s=w519, f=w520) -> (s? t:f=→"Dp_error_dd":fxp<+/-,41,26>)
  }
  n310 = while "Omega_p(T method)" {
    shift-right: [w556] -> _
    shift-left: _ -> [w554]
    shift-right: [w537] -> _
    shift-left: _ -> [w555]
    shift-right: [w552] -> _
    shift-left: _ -> [w553]
    shift-right: [w530] -> _
    shift-left: _ -> [w529]
    shift-right: [w525] -> _
    shift-left: _ -> [w527]
    shift-right: [w533] -> _
    shift-left: _ -> [w532]
    stop <- FALSE stop-if-true
    w544 = fxp<+/-,32,0> 0.3183098859153688  # L/2/pi
    w549 = fxp<+/-,32,0> 0.3183098859153688  # L/2/pi
    n311 = local read "Encoder Position_p1"() -> (w556:i32)
    n312 = local read "Encoder Position_p2"() -> (w530:i32)
    n313 = call "Tick Count4"() -> ("Tick Count(Ticks)"=w531:u32)
    n314 = call "omega_sub_Encoder_800ppr.vi"("mt0"="mt0_p1", "omega_pre"=w555, "ticks_m_pre"=w553, "ticks"=w531, "count_pre"=w554, "count"=w556) -> ("ticks_m"=w552:u32, "mt"=→"mt_omega_p1":u32, "omega"=w537:fxp<+/-,36,13>)  [unwired: 3 in]
    "omega_p1 (T)" <- w537
    n315 = call "omega_sub_Encoder_4096ppr.vi"("mt0"="mt0_p2", "omega_pre"=w527, "ticks_m_pre"=w532, "ticks"=w531, "count_pre"=w529, "count"=w530) -> ("ticks_m"=w533:u32, "mt"=→"mt_omega_p2":u32, "omega"=w525:fxp<+/-,36,13>)  [unwired: 3 in]
    n316 = local read "Mag. factor_p"() -> (w545:fxp<+/-,20,3>)
    n317 = local read "Belt_in_p"() -> (w542:fxp<+/-,6,6>)
    n318 = local read "Belt_out_p"() -> (w541:fxp<+/-,7,7>)
    n319 = Multiply(x=w549, y="Belt_in_p") -> (x*y=w547:fxp<+/-,38,6>)
    n320 = Multiply(x=w544, y=w542) -> (x*y=w543:fxp<+/-,38,6>)
    n321 = Divide(x=w547, y="Belt_out_p") -> (x/y=w538:fxp<+/-,20,1>)
    n322 = Divide(x=w525, y=w545) -> (x/y=w526:fxp<+/-,57,31>)
    "omega_p2 (T)" <- w526
    n323 = Divide(x=w543, y=w541) -> (x/y=w536:fxp<+/-,45,6>)
    n324 = Multiply(x=w536, y=w526) -> (x*y=→"Dp2_d (T)":fxp<+/-,36,13>)
    n325 = Multiply(x=w538, y=w537) -> (x*y=→"Dp1_d (T)":fxp<+/-,36,13>)
  }
  n326 = while {
    tunnel: [w557] -> w9
    shift-right: [w581] -> _
    shift-left: _ -> [w582]
    tunnel: w16 -> [w577]
    shift-right: [w573] -> _
    shift-left: _ -> [w574]
    shift-right: [w569] -> _
    shift-left: _ -> [w568]
    shift-right: [w568] -> _
    shift-left: _ -> [w567]
    shift-right: [w567] -> _
    shift-left: _ -> [w566]
    shift-right: [w566] -> _
    shift-left: _ -> [w565]
    shift-right: [w565] -> _
    shift-left: _ -> [w564]
    shift-right: [w564] -> _
    shift-left: _ -> [w563]
    shift-right: [w563] -> _
    shift-left: _ -> [w562]
    stop <- w576 stop-if-true
    w571 = fxp<+,20,2> 2.115001678466797  # Gage Factor
    n327 = xnode "FPGA I/O Node"("error in"=w577) -> ("error out"=w557:errorcluster, "Mod6/AI3"=w572:fxp<+/-,24,-4>)  [unwired: 1 in, 1 out]
    n328 = Select(t=w572, s="Strain gage reset_p", f=w574) -> (s? t:f=w573:fxp<+/-,24,-4>)
    n329 = Or(x="Stop (Strain)", y=w557) -> (x .or. y?=w576:bool)
    n330 = Subtract(x=w572, y=w573) -> (x-y=w570:fxp<+/-,30,-3>)
    "Mod6/AI3" <- w570
    n331 = Multiply(x=w571, y=w570) -> (x*y=w569:fxp<+/-,50,-1>)
    "Raw Strain_p" <- w569
    n332 = call "average_v2.vi"("Numeric 8"=w562, "Numeric"=w569, "Numeric 7"=w563, "Numeric 2"=w568, "Numeric 6"=w564, "Numeric 5"=w565, "Numeric 4"=w566, "Numeric 3"=w567) -> ("Mean (8pt)"=w561:fxp<+/-,32,4>)  [unwired: 1 in, 2 out]
    "Strain_p (Avg8)" <- w561
    n333 = call "Tick Count"() -> ("Tick Count(uSec)"=w581:u32)
    n334 = xnode "Butterworth Filter"("input data"=w561, "scaled coefficients"="Strain_p Avg.8 coeff.") -> ("output data"=→"Strain_p (Avg8 w. f)":fxp<+/-,36,8>)  [unwired: 1 in]
    n335 = Subtract(x=w581, y=w582) -> (x-y=w580:fxp<+/-,32,16>)
    n336 = Divide(x=fxp<+,7,10> 1000.0, y=w580) -> (x/y=→"Loop rate (kHz)":fxp<+/-,40,27>)
  }
  n337 = while {
    stop <- FALSE stop-if-true
    n338 = local read "omega_p1 (Mavg)"() -> (w598:fxp<+/-,36,14>)
    n339 = local read "Dp1_d (Mavg)"() -> (w594:fxp<+/-,36,14>)
    n340 = call "Loop Timer2"("Count(uSec)"="Mavg f loop(uSec)") -> ()  [unwired: 1 out]
    n341 = xnode "Butterworth Filter"("input data"=w598, "scaled coefficients"="omega_P(Mavg) coeff.") -> ("output data"=→"omega_p (Mavg w. f)":fxp<+/-,36,18>)  [unwired: 1 in]
    n342 = xnode "Butterworth Filter"("input data"=w594, "scaled coefficients"="Dp_d (Mavg) coeff.") -> ("output data"=→"Dp_d (Mavg w. f.)":fxp<+/-,36,18>)  [unwired: 1 in]
  }
  n343 = while "Quadrature drive_p" {
    stop <- FALSE stop-if-true
    n344 = local read "Drive mode"() -> (w616:i16)
    n345 = case shown="2" w616 {
      tunnel: [w626 w627 w628] -> w615
      frame 0, Default {
        # "Backward"
        n346 = local read "Fp_PID"() -> (w626:fxp<+/-,36,16>)
      }
      frame 1 {
        # "Forward"
        n347 = local read "Fr_p"() -> (w627:fxp<+/-,32,10>)
      }
      frame 2 {
        # "Imp"
        n348 = local read "Fp_PID"() -> (w628:fxp<+/-,36,16>)
      }
    }
    n349 = local read "dFp_PID"() -> (w619:fxp<+/-,36,18>)
    n350 = local read "omega_p (rad/s)"() -> (w623:fxp<+/-,36,13>)
    n351 = Select(t=w619, s="dFp_add", f=fxp<+,1,1> 0.0) -> (s? t:f=w622:fxp<+/-,36,18>)
    n352 = call "Oriental_step_motor_PKP225.vi"("F_Threshold"="F_Threshold_p", "dFmr"=w622, "omega"=w623, "Fmr"=w615) -> ("vq_F"=→"vq_p_F":fxp<+/-,36,9>, "vd_F"=→"vd_p_F":fxp<+/-,36,9>)  [unwired: 6 in]
  }
  n353 = xnode "FPGA I/O Node"("error in"=w9, "Mod6/Stop"=TRUE) -> ()  [unwired: 1 in, 2 out]
